vi "Reset.vi"(8 "error in (no error)":errorcluster, 11 "VISA resource name":refnum<visa-resource-name>) -> (0 "error out":errorcluster, 3 "VISA resource name out":refnum<visa-resource-name>)   [LabVIEW 2013, in "HadCon.lvlib"]
doc: "Resets the instrument and then sends a set of default setup commands to the instrument."
uses:
  <instrlib>/HadCon/HadCon.lvlib
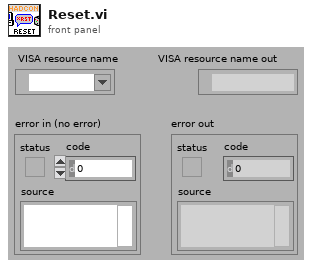
[diagram p1: front panel]
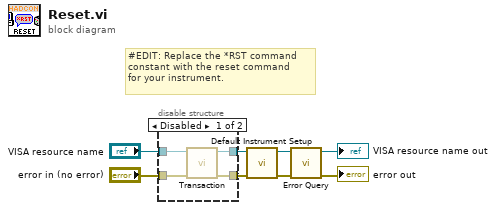
[diagram p0: block diagram]
diagram:
  # "#EDIT: Replace the *RST command\nconstant with the reset command\nfor your instrument."
  n1 = disable-structure shown="Disabled" {
    disable-tunnel: "VISA resource name" -> [w12 w14]
    disable-tunnel: [w11 w14] -> w3
    disable-tunnel: "error in (no error)" -> [w10 w13]
    disable-tunnel: [w9 w13] -> w1
    frame Disabled {
      n2 = call <instrlib>:"Transaction.vi"("Error In"=w10, "VISA resource name"=w12) -> ("Error Out"=w9:errorcluster, "VISA resource name out"=w11:refnum<visa-resource-name>)  [unwired: 7 in, 1 out]
    }
    frame Enabled {
    }
  }
  n3 = call <instrlib>:"Default Instrument Setup.vi"("error in (no error)"=w1, "VISA resource name"=w3) -> ("error out"=w8:errorcluster, "VISA resource name out"=w7:refnum<visa-resource-name>)  [unwired: 8 in]
  n4 = call <instrlib>:"Error Query.vi"("error in (no error)"=w8, "VISA resource name"=w7) -> ("error out"=→"error out":errorcluster, "VISA resource name out"=→"VISA resource name out":refnum<visa-resource-name>)  [unwired: 6 in, 2 out]
